vi "Cont Acq - Ch Expansion Sync - External Clock.vi"() -> ()   [LabVIEW 2026]
uses:
  <vilib>/DAQmx/read.llb/DAQmx Read (Analog 1D Wfm NChan NSamp).vi
  <vilib>/FPGAPlugInAG/PXIe-7856R/niLvFpga_Open_PXIe-7856R.vi
  <vilib>/rvi/interface/common/dynamic/niFpgaDynamicAddResources.vi
  <vilib>/Utility/error.llb/Error Cluster From Error Code.vi
  <vilib>/rvi/errors/niLvFpgaAdjustHostInterfaceError.vi
  <vilib>/FPGAPlugInAG/Dynamic/niLvFpga_Run_Dynamic.vi
  <vilib>/DAQmx/create/channels.llb/DAQmx Create Channel (AI-Voltage-Basic).vi
  <vilib>/DAQmx/configure/timing.llb/DAQmx Timing (Sample Clock).vi
  <vilib>/DAQmx/miscellaneous.llb/DAQmx Fill In Error Info.vi
  <vilib>/FPGAPlugInAG/Dynamic/niLvFpga_Close_Dynamic.vi
  <vilib>/rvi/interface/nirviOpenFPGA/nirviOpenFPGA.xnode
  FPGA Bitfiles/PulseAndClockGeneration.lvbitx
  FPGA/Pulse and Clock Generation.vi
  <vilib>/rvi/interface/nirviReadWriteControl/nirviReadWriteControl.xnode
  <vilib>/rvi/interface/nirviMethod/nirviMethod.xnode
  <vilib>/rvi/interface/nirviCloseFPGA/nirviCloseFPGA.xnode
  <vilib>/rvi/interface/Simulation/niFpgaSimulationCallBeginRW.vi
  NiFpgaLv.dll
panel:
  out "Calculated Sample Rate":dbl format="%#_2p"
  out "Samples":i32
  out "Timing Chart":u32(graph)
  out "Iteration Time (ms)":u32
  in  "stop":bool
  out "Waveform Graph":waveform(dbl)[](graph)
  out "error out":errorcluster
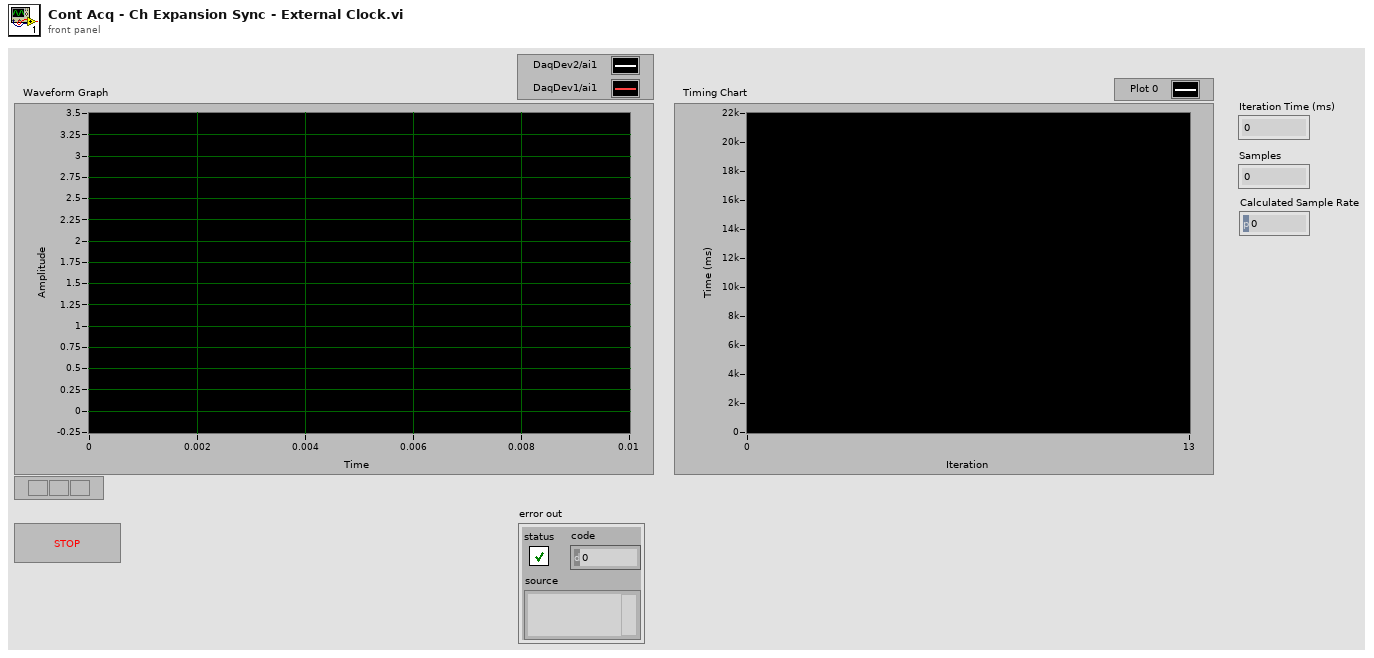
[diagram p1: front panel]
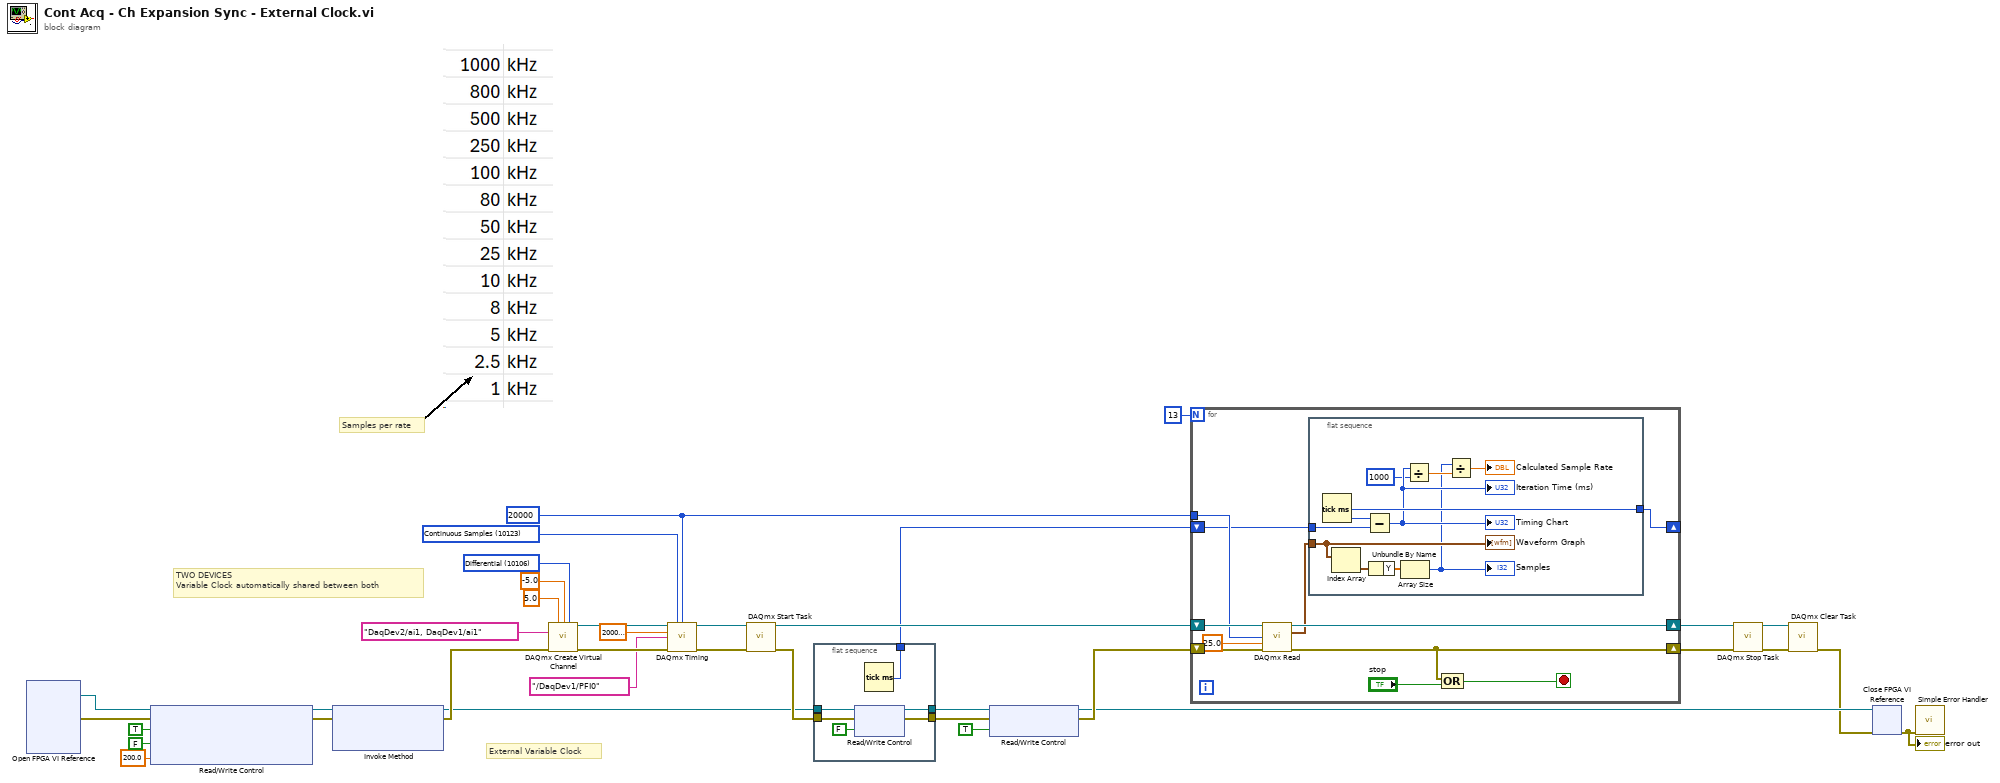
[diagram p0: block diagram]
diagram:
  w5 = 20000 ("number of samples per channel")
  w30 = 10123 items=["Finite Samples"=10178, "Continuous Samples"=10123, "Hardware Timed Single Point"=12522] ("sample mode")
  w35 = 10106 items=["Default"=-1, "RSE"=10083, "NRSE"=10078, "Differential"=10106, "Pseudodifferential"=12529] ("input terminal configuration")
  # "Samples per rate"
  # "External Variable Clock"
  # "TWO DEVICES\nVariable Clock automatically shared between both"
  n1 = xnode "Open FPGA VI Reference"() -> ("FPGA VI Reference Out"=w24:refnum<k20>, "error out"=w23:errorcluster)  [unwired: 2 in]
  n2 = xnode "Read/Write Control"("FPGA VI Reference In"=w24, "error in"=w23, "Reset"=TRUE, "Enable Output"=FALSE ("Connector1/DIO0"), "Requested Output Frequency"=sgl 200.0 ("Requested Clock frequency")) -> ("FPGA VI Reference Out"=w22:refnum<k20>, "error out"=w21:errorcluster)
  n3 = xnode "Invoke Method"("FPGA VI Reference In"=w22, "error in"=w21) -> ("FPGA VI Reference Out"=w11:refnum<k20>, "error out"=w20:errorcluster)  [unwired: 1 in]
  n4 = call-poly <vilib>:"DAQmx Create Virtual Channel.vi"("maximum value"=5.0, "minimum value"=-5.0, "input terminal configuration"=w35, "physical channels"=tag "DaqDev2/ai1, DaqDev1/ai1", "error in"=w20) -> ("task out"=w32:refnum<k21>, "error out"=w31:errorcluster)  [unwired: 9 in]
  n5 = call-poly <vilib>:"DAQmx Timing.vi"("task/channels in"=w32, "sample mode"=w30, "samples per channel"=w5, "rate"=2000000.0, "source"=tag "/DaqDev1/PFI0", "error in"=w31) -> ("task out"=w3:refnum<k21>, "error out"=w4:errorcluster)  [unwired: 8 in]
  n6 = call <vilib>:"DAQmx Start Task.vi"("task/channels in"=w3, "error in"=w4) -> ("task out"=w29:refnum<k21>, "error out"=w12:errorcluster)  [unwired: 12 in]
  n7 = flat-sequence {
    tunnel: w12 -> [w42]
    tunnel: w11 -> [w41]
    tunnel: [w40] -> w10
    tunnel: [w38] -> w7
    tunnel: [w37] -> w2
    frame #0 {
      n8 = xnode "Read/Write Control"("FPGA VI Reference In"=w41, "error in"=w42, "Reset"=FALSE ("Trigger")) -> ("FPGA VI Reference Out"=w40:refnum<k20>, "error out"=w38:errorcluster)
      n9 = Tick Count (ms)() -> (millisecond timer value=w37:u32)
    }
  }
  n10 = xnode "Read/Write Control"("FPGA VI Reference In"=w10, "error in"=w7, "Enable Output"=TRUE ("Connector1/DIO0")) -> ("FPGA VI Reference Out"=w18:refnum<k20>, "error out"=w19:errorcluster)
  n11 = for {
    N: 13 -> [_]
    shift-right: [w52] -> w28
    shift-left: w29 -> [w53]
    shift-right: [w48] -> w26
    shift-left: w19 -> [w51]
    tunnel: w5 -> [w47]
    shift-right: [w45] -> _
    shift-left: w2 -> [w46]
    stop <- w44 stop-if-true
    n12 = call-poly <vilib>:"DAQmx Read.vi"("task/channels in"=w53, "number of samples per channel"=w47, "timeout"=25.0, "error in"=w51) -> ("task out"=w52:refnum<k21>, "data"=w50:waveform(dbl)[], "error out"=w48:errorcluster)  [unwired: 9 in]
    n13 = flat-sequence {
      tunnel: w50 -> [w61]
      tunnel: w46 -> [w62]
      tunnel: [w63] -> w45
      frame #0 {
        n14 = Tick Count (ms)() -> (millisecond timer value=w63:u32)
        n15 = Index Array(array=w61) -> (element=w60:waveform(dbl))  [unwired: 1 in]
        n16 = Subtract(x=w63, y=w62) -> (x-y=w58:u32)
        "Iteration Time (ms)" <- w58
        "Timing Chart" <- w58
        n17 = Unbundle By Name(w60) -> ("Y"=w59:dbl[])
        n18 = Array Size(array=w59) -> (size(s)=w55:i32)
        "Samples" <- w55
        n19 = Divide(x=w58, y=u32 1000) -> (x/y=w56:dbl)
        n20 = Divide(x=w55, y=w56) -> (x/y=→"Calculated Sample Rate":dbl)
        "Waveform Graph" <- w61
      }
    }
    n21 = Compound Arithmetic op=OR(w48, "stop") -> (w44:bool)
  }
  n22 = call <vilib>:"DAQmx Stop Task.vi"("task/channels in"=w28, "error in"=w26) -> ("task out"=w27:refnum<k21>, "error out"=w25:errorcluster)  [unwired: 12 in]
  n23 = call <vilib>:"DAQmx Clear Task.vi"("task in"=w27, "error in"=w25) -> ("error out"=w17:errorcluster)  [unwired: 13 in]
  n24 = xnode "Close FPGA VI Reference"("FPGA VI Reference In"=w18, "error in"=w17) -> ("error out"=w16:errorcluster)
  "error out" <- w16
  n25 = call <vilib>:"Simple Error Handler.vi"("error in (no error)"=w16) -> ()  [unwired: 4 in, 5 out]
